vi "io_attr_query.vi"(5 "Query Parameter (None)":string, 7 "Attribute":T1={"Identifier"="", "Descriptive Name"="", "Data Type"=enum."Integer 32", "Command"="", "Access"=enum."Read/Write", "Range Table"="", "Read Callback"="", "Write Callback"="", "Supported Models"="", "Instrument Options"="", "Index"=0, "OPC Wait"=FALSE, "No Status Check"=FALSE, "Cache Only"=FALSE}, 8 "error in":errorcluster caption="error in (no error)", 10 "write buffer":string, 11 "VISA resource name":refnum<visa-resource-name>) -> (0 "error out":errorcluster, 2 "read buffer":string, 3 "VISA resource name out":refnum<visa-resource-name>)   [LabVIEW 2020, in "Rohde&Schwarz RTx Oscilloscopes.lvlib" / "rsidr_core.lvlib"]
uses:
  rsidr_core.lvlib
  type_Attribute.ctl
  type_Attribute_Data_Type.ctl
  type_ReadWriteAccess.ctl
  _type_Operation_Fgv_RangeTable.ctl
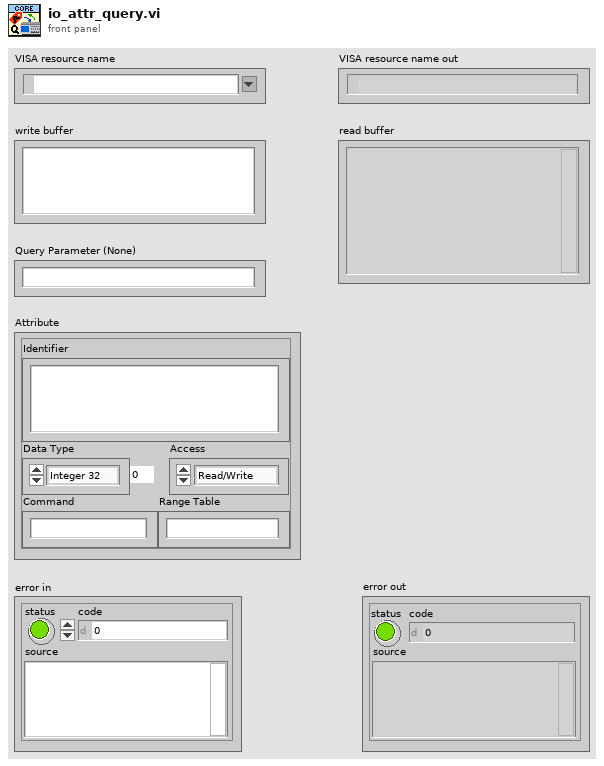
[diagram p1: front panel]
types:
  T1 = typedef "Rohde&Schwarz RTx Oscilloscopes.lvlib/rsidr_core.lvlib/type_Attribute.ctl" = cluster{"Identifier":string, "Descriptive Name":string, "Data Type":T2, "Command":string, "Access":T3, "Range Table":string, "Read Callback":string, "Write Callback":string, "Supported Models":string, "Instrument Options":string, "Index":i32, "OPC Wait":bool, "No Status Check":bool, "Cache Only":bool}
  T2 = typedef "Rohde&Schwarz RTx Oscilloscopes.lvlib/rsidr_core.lvlib/type_Attribute_Data_Type.ctl" = enum16{"Integer 32", "Double", "String", "Boolean", "None", "Integer 64", "RawString"}
  T3 = typedef "Rohde&Schwarz RTx Oscilloscopes.lvlib/rsidr_core.lvlib/type_ReadWriteAccess.ctl" = enum16{"Read Only", "Write Only", "Read/Write"}
  T4 = typedef "Rohde&Schwarz RTx Oscilloscopes.lvlib/rsidr_core.lvlib/_type_Operation_Fgv_RangeTable.ctl" = enum16{"Initialize", "Check", "Coerce", "Get Command String", "Get Numeric Value", "Get Default Value", "Get Range Table Type"}
  T5 = typedef "Rohde&Schwarz RTx Oscilloscopes.lvlib/rsidr_core.lvlib/type_Session_Data.ctl" = cluster{"IDN string":string, "Instrument FW":string, "Instr type":string, "Instr type for err. msg.":string, "Installed Options":string[], "Ignore Error Messages":string, "Logging params":variant, "OPC Timeout":i32, "VISA Timeout":i32, "STB Poll VISA Timeout":i32, "Additional Flags":i32, "Wait Before Read":i32, "Wait Before Write":i32, "Option String Flags":i32, "IO Segment Size":i64, "VISA Access Mode":T6, "Interface Type":T7, "OPC Wait Mode":T8, "Bin Float Number  Format":T9, "Bin Integer Number Format":T10, "Simulate":bool, "VXIcapable":bool, "Duplicate Session":bool, "Add LF to Write":bool, "Logging":bool, "Fast Sweep":bool, "Query Instrument Status":bool, "Check Range":bool, "Check Options":bool, "OPC-sync Attr Writes":bool, "OPC-sync Attr Queries":bool}
  T6 = typedef "Rohde&Schwarz RTx Oscilloscopes.lvlib/rsidr_core.lvlib/type_VisaAccessMode.ctl" = u16
  T7 = typedef "Rohde&Schwarz RTx Oscilloscopes.lvlib/rsidr_core.lvlib/type_InterfaceType.ctl" = enum16{"Unknown", "GPIB", "VXI", "GPIB_VXI", "ASRL", "PXI", "TCPIP", "USB", "SOCKET"}
  T8 = typedef "Rohde&Schwarz RTx Oscilloscopes.lvlib/rsidr_core.lvlib/type_OPC_Wait_Mode.ctl" = enum16{"STBpolling", "STBpollingSlow", "STBpollingSuperSlow", "ServiceRequest", "OPCquery"}
  T9 = typedef "Rohde&Schwarz RTx Oscilloscopes.lvlib/rsidr_core.lvlib/type_Binary_Float_Number_Format.ctl" = enum16{"Float_4_Bytes_Swapped", "Float_4_Bytes", "Double_8_Bytes_Swapped", "Double_8_Bytes"}
  T10 = typedef "Rohde&Schwarz RTx Oscilloscopes.lvlib/rsidr_core.lvlib/type_Binary_Integer_Number_Format.ctl" = enum16{"Int32_4_Bytes_Swapped", "Int32_4 Bytes", "Int16_2_Bytes_Swapped", "Int16_2_Bytes"}
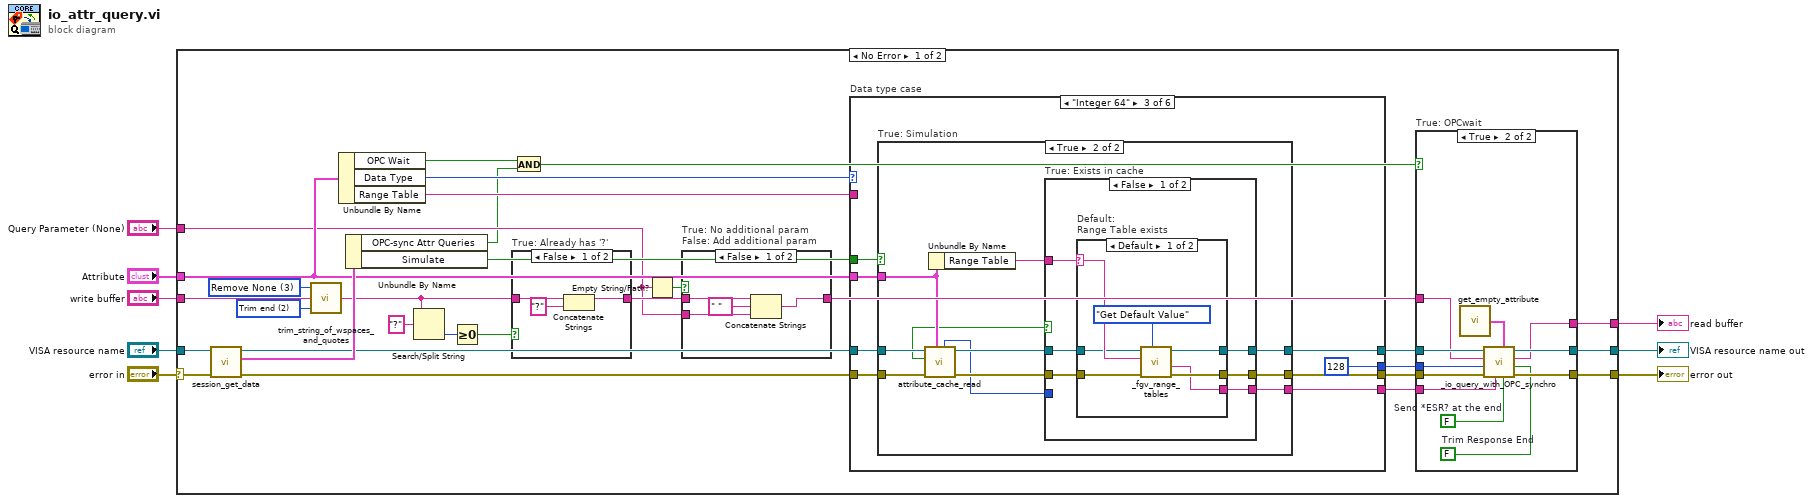
[diagram p0: block diagram]
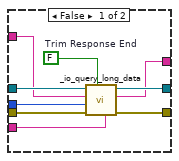
[diagram p3: hidden frame]
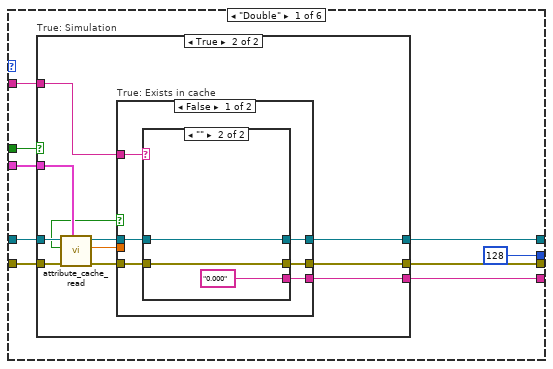
[diagram p5: hidden frame]
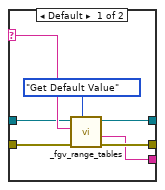
[diagram p7: hidden frame]
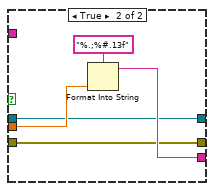
[diagram p8: hidden frame]
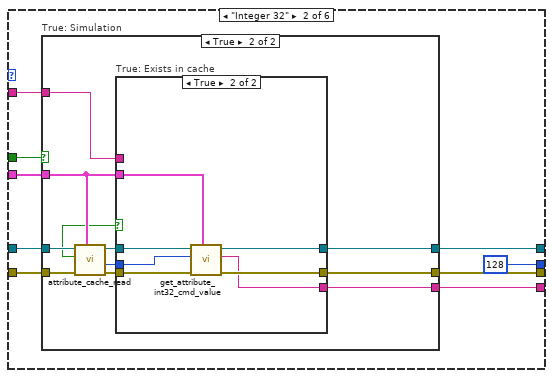
[diagram p9: hidden frame]
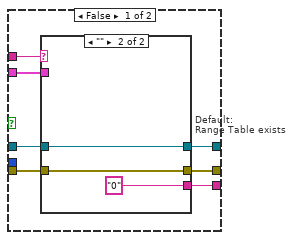
[diagram p11: hidden frame]
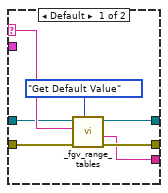
[diagram p12: hidden frame]
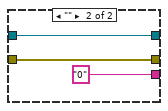
[diagram p14: hidden frame]
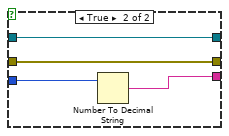
[diagram p15: hidden frame]
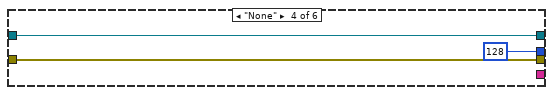
[diagram p16: hidden frame]
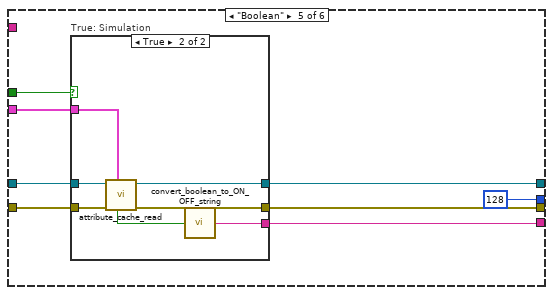
[diagram p17: hidden frame]
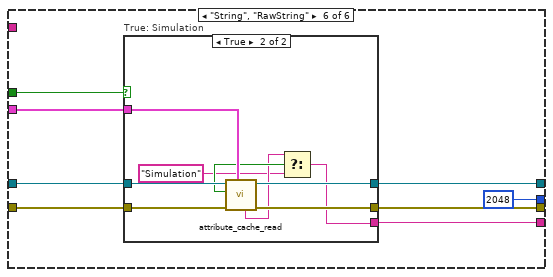
[diagram p19: hidden frame]
diagram:
  n1 = case shown="No Error" "error in" {
    selector: "error in" -> [w35 w238]
    tunnel: "VISA resource name" -> [w34 w237]
    tunnel: [w20 w238] -> w3
    tunnel: [w19 w237] -> w2
    tunnel: [w16 _] -> w8
    tunnel: "write buffer" -> [w28 _]
    tunnel: "Attribute" -> [w33 _]
    tunnel: "Query Parameter (None)" -> [w13 _]
    frame No Error {
      w25 = u16 3 items=["Remove All Quotes", "Remove Single Quotes", "Remove Double Quotes", "Remove None"] ("Remove quotes (Remove All)")
      w27 = u16 2 items=["Trim both", "Trim start", "Trim end", "Trim none"] ("Trim whitespaces (Trim both)")
      n2 = call "session_get_data.vi"("error in"=w35, "VISA resource name"=w34) -> ("error out"=w23:errorcluster, "Session User Data out"=w38:T5, "VISA resource name out"=w24:refnum<visa-resource-name>)  [unwired: 6 in, 1 out]
      n3 = call "trim_string_of_wspaces_and_quotes.vi"("Trim whitespaces (Trim both)"=w27, "String in"=w28, "Remove quotes (Remove All)"=w25) -> ("String out"=w26:string)  [unwired: 2 in]
      n4 = Unbundle By Name(w33) -> ("OPC Wait"=w11:bool, "Data Type"=w37:T2, "Range Table"=w29:string)
      n5 = Unbundle By Name(w38) -> ("OPC-sync Attr Queries"=w10:bool, "Simulate"=w36:bool)
      n6 = Search/Split String(string=w26, search string/char (-)="?" ("string")) -> (offset of match=w31:i32)  [unwired: 1 in, 2 out]
      n7 = Greater Or Equal To 0?(x=w31) -> (x >= 0?=w30:bool)
      n8 = case "True: Already has '?'" shown="False" w30 {
        tunnel: w26 -> [w66 w67]
        tunnel: [w64 w67] -> w14
        frame False {
          n9 = Concatenate Strings(w66, "?" ("string")) -> (w64:string)
        }
        frame True {
        }
      }
      n10 = And(x=w11, y=w10) -> (x .and. y?=w9:bool)
      n11 = Empty String/Path?(string/path=w13) -> (empty?=w15:bool)
      n12 = case "True: No additional param\nFalse: Add additional param" shown="False" w15 {
        tunnel: w14 -> [w40 w43]
        tunnel: [w39 w43] -> w12
        tunnel: w13 -> [w41 _]
        frame False {
          n13 = Concatenate Strings(w40, " " ("string"), w41) -> (w39:string)
        }
        frame True {
        }
      }
      n14 = case "Data type case" shown="\"Integer 64\"" w37 {
        tunnel: w23 -> [w75 w118 w162 w199 w207 w224]
        tunnel: w24 -> [w74 w117 w161 w200 w206 w223]
        tunnel: [w69 w113 w159 w199 w203 w220] -> w22
        tunnel: [w70 w114 w160 w200 w204 w221] -> w21
        tunnel: w36 -> [w76 w119 w163 _ w208 w225]
        tunnel: w33 -> [w73 w115 w164 _ w205 w222]
        tunnel: w29 -> [w72 w116 _ _ _ _]
        tunnel: [w71 w112 w158 _ w202 w219] -> w18
        tunnel: [u32 128 u32 128 u32 128 u32 128 u32 128 u32 2048] -> w17
        frame "Double" {
          n15 = case "True: Simulation" shown="True" w76 {
            tunnel: w75 -> [w78 w89]
            tunnel: w74 -> [w77 w88]
            tunnel: [w77 w81] -> w70
            tunnel: [w78 w85] -> w69
            tunnel: w73 -> [_ w84]
            tunnel: [_ w79] -> w71
            tunnel: w72 -> [_ w80]
            frame False {
            }
            frame True {
              n16 = call "attribute_cache_read.vi"("Attribute"=w84, "error in"=w89, "VISA resource name"=w88) -> ("error out"=w87:errorcluster, "Double out"=w86:dbl, "VISA resource name out"=w82:refnum<visa-resource-name>, "Exists in cache"=w83:bool)  [unwired: 1 in, 4 out]
              n17 = case "True: Exists in cache" shown="False" w83 {
                tunnel: w87 -> [w93 w107]
                tunnel: w86 -> [_ w108]
                tunnel: [w92 w107] -> w85
                tunnel: [w94 w109] -> w79
                tunnel: w80 -> [w95 _]
                tunnel: w82 -> [w91 w106]
                tunnel: [w90 w106] -> w81
                frame False {
                  n18 = case shown="\"\"" w95 {
                    selector: w95 -> [w100 _]
                    tunnel: [w96 "0.000"] -> w94
                    tunnel: w93 -> [w102 w104]
                    tunnel: [w101 w104] -> w92
                    tunnel: w91 -> [w99 w103]
                    tunnel: [w98 w103] -> w90
                    frame Default {
                      n19 = call "_fgv_range_tables.vi"("Operation"=_type_Operation_Fgv_RangeTable."Get Default Value", "error in"=w102, "Range Table ID in"=w100, "VISA resource name"=w99) -> ("error out"=w101:errorcluster, "String Value out"=w96:string, "VISA resource name out"=w98:refnum<visa-resource-name>)  [unwired: 3 in, 2 out]
                    }
                    frame "" {
                    }
                  }
                }
                frame True {
                  n20 = Format Into String(format string="%.;%#.13f", w108) -> (resulting string=w109:string)  [unwired: 2 in, 1 out]
                }
              }
            }
          }
        }
        frame "Integer 32" {
          n21 = case "True: Simulation" shown="True" w119 {
            tunnel: w118 -> [w121 w132]
            tunnel: w117 -> [w120 w131]
            tunnel: [w120 w124] -> w114
            tunnel: [w121 w129] -> w113
            tunnel: w115 -> [_ w130]
            tunnel: [_ w122] -> w112
            tunnel: w116 -> [_ w123]
            frame False {
            }
            frame True {
              n22 = call "attribute_cache_read.vi"("Attribute"=w130, "error in"=w132, "VISA resource name"=w131) -> ("error out"=w127:errorcluster, "Int32 out"=w128:i32, "VISA resource name out"=w125:refnum<visa-resource-name>, "Exists in cache"=w126:bool)  [unwired: 1 in, 4 out]
              n23 = case "True: Exists in cache" shown="True" w126 {
                tunnel: w123 -> [w139 _]
                tunnel: w130 -> [w138 w151]
                tunnel: [w137 w154] -> w129
                tunnel: w128 -> [_ w152]
                tunnel: w127 -> [w136 w156]
                tunnel: w125 -> [w135 w155]
                tunnel: [w134 w153] -> w124
                tunnel: [w133 w150] -> w122
                frame False {
                  n24 = case "Default:\nRange Table exists" shown="\"\"" w139 {
                    selector: w139 -> [w144 _]
                    tunnel: [w145 w149] -> w137
                    tunnel: w138 -> [_ _]
                    tunnel: w136 -> [w146 w149]
                    tunnel: w135 -> [w143 w148]
                    tunnel: [w142 w148] -> w134
                    tunnel: [w140 "0" ("String Value out")] -> w133
                    frame Default {
                      n25 = call "_fgv_range_tables.vi"("Operation"=_type_Operation_Fgv_RangeTable."Get Default Value", "error in"=w146, "Range Table ID in"=w144, "VISA resource name"=w143) -> ("error out"=w145:errorcluster, "String Value out"=w140:string, "VISA resource name out"=w142:refnum<visa-resource-name>)  [unwired: 3 in, 2 out]
                    }
                    frame "" {
                    }
                  }
                }
                frame True {
                  n26 = call "get_attribute_int32_cmd_value.vi"("Attribute"=w151, "error in"=w156, "Input Int32 value"=w152, "VISA resource name"=w155) -> ("error out"=w154:errorcluster, "Cmd Value out"=w150:string, "VISA resource name out"=w153:refnum<visa-resource-name>)  [unwired: 5 in]
                }
              }
            }
          }
        }
        frame "Integer 64" {
          n27 = case "True: Simulation" shown="True" w163 {
            tunnel: w162 -> [w166 w177]
            tunnel: w161 -> [w165 w176]
            tunnel: [w165 w169] -> w160
            tunnel: [w166 w173] -> w159
            tunnel: w164 -> [_ w174]
            tunnel: [_ w168] -> w158
            frame False {
            }
            frame True {
              n28 = call "attribute_cache_read.vi"("Attribute"=w174, "error in"=w177, "VISA resource name"=w176) -> ("error out"=w172:errorcluster, "VISA resource name out"=w170:refnum<visa-resource-name>, "Int64 out"=w167:i64, "Exists in cache"=w171:bool)  [unwired: 1 in, 4 out]
              n29 = Unbundle By Name(w174) -> ("Range Table"=w175:string)
              n30 = case "True: Exists in cache" shown="False" w171 {
                tunnel: w175 -> [w183 _]
                tunnel: [w182 w196] -> w173
                tunnel: [w181 w197] -> w168
                tunnel: w167 -> [_ w194]
                tunnel: w172 -> [w180 w196]
                tunnel: w170 -> [w179 w195]
                tunnel: [w178 w195] -> w169
                frame False {
                  n31 = case "Default:\nRange Table exists" shown="Default" w183 {
                    selector: w183 -> [w188 _]
                    tunnel: [w189 w193] -> w182
                    tunnel: [w184 "0"] -> w181
                    tunnel: w180 -> [w190 w193]
                    tunnel: w179 -> [w187 w191]
                    tunnel: [w186 w191] -> w178
                    frame Default {
                      n32 = call "_fgv_range_tables.vi"("Operation"=_type_Operation_Fgv_RangeTable."Get Default Value", "error in"=w190, "Range Table ID in"=w188, "VISA resource name"=w187) -> ("error out"=w189:errorcluster, "String Value out"=w184:string, "VISA resource name out"=w186:refnum<visa-resource-name>)  [unwired: 3 in, 2 out]
                    }
                    frame "" {
                    }
                  }
                }
                frame True {
                  n33 = Number To Decimal String(number=w194) -> (decimal integer string=w197:string)  [unwired: 1 in]
                }
              }
            }
          }
        }
        frame "None" {
        }
        frame "Boolean" {
          n34 = case "True: Simulation" shown="True" w208 {
            tunnel: w207 -> [w210 w217]
            tunnel: w206 -> [w209 w216]
            tunnel: [w209 w215] -> w204
            tunnel: [w210 w213] -> w203
            tunnel: w205 -> [_ w214]
            tunnel: [_ w211] -> w202
            frame False {
            }
            frame True {
              n35 = call "attribute_cache_read.vi"("Attribute"=w214, "error in"=w217, "VISA resource name"=w216) -> ("error out"=w213:errorcluster, "VISA resource name out"=w215:refnum<visa-resource-name>, "Boolean out"=w212:bool)  [unwired: 1 in, 5 out]
              n36 = call "convert_boolean_to_ON_OFF_string.vi"("boolean value in"=w212) -> ("string value out"=w211:string)  [unwired: 4 in]
            }
          }
        }
        frame "String", "RawString" {
          n37 = case "True: Simulation" shown="True" w225 {
            tunnel: w224 -> [w227 w236]
            tunnel: w223 -> [w226 w235]
            tunnel: [w226 w234] -> w221
            tunnel: [w227 w232] -> w220
            tunnel: w222 -> [_ w233]
            tunnel: [_ w231] -> w219
            frame False {
            }
            frame True {
              n38 = call "attribute_cache_read.vi"("Attribute"=w233, "error in"=w236, "VISA resource name"=w235) -> ("error out"=w232:errorcluster, "VISA resource name out"=w234:refnum<visa-resource-name>, "String out"=w229:string, "Exists in cache"=w230:bool)  [unwired: 1 in, 4 out]
              n39 = Select(t=w229, s=w230, f="Simulation") -> (s? t:f=w231:string)
            }
          }
        }
      }
      n40 = case "True: OPCwait" shown="True" w9 {
        tunnel: w22 -> [w52 w63]
        tunnel: w21 -> [w51 w62]
        tunnel: [w50 w61] -> w20
        tunnel: [w49 w60] -> w19
        tunnel: w12 -> [w47 w55]
        tunnel: w18 -> [w45 w56]
        tunnel: w17 -> [w48 w59]
        tunnel: [w46 w58] -> w16
        frame False {
          w44 = FALSE  # Trim Response End
          n41 = call "_io_query_long_data.vi"("Simulation read buffer (\"Simulation\")"=w45, "Trim Response End"=w44, "error in"=w52, "Max chunk read bytes count (65536)"=w48, "Write buffer"=w47, "VISA resource name"=w51) -> ("error out"=w50:errorcluster, "Read buffer"=w46:string, "VISA resource name out"=w49:refnum<visa-resource-name>)  [unwired: 3 in]
        }
        frame True {
          w54 = FALSE  # Trim Response End
          w57 = FALSE  # Send *ESR? at the end
          n42 = call "get_empty_attribute.vi"() -> ("Empty Attribute out"=w53:T1)
          n43 = call "_io_query_with_OPC_synchro.vi"("Trim Response End"=w54, "Send *ESR? at the end (T)"=w57, "Attribute"=w53, "Simulation read buffer (\"Simulation\")"=w56, "error in"=w63, "Max segment read bytes count (65536)"=w59, "Query"=w55, "VISA resource name"=w62) -> ("error out"=w61:errorcluster, "Response"=w58:string, "VISA resource name out"=w60:refnum<visa-resource-name>)  [unwired: 1 in]
        }
      }
    }
    frame Error {
    }
  }
  "VISA resource name out" <- w2
  "error out" <- w3
  "read buffer" <- w8
